vi "Global_Sensors.vi"() -> ()   [LabVIEW 2018]
panel:
  in  "Distance Along Path":dbl
  out "Sensor 1":bool
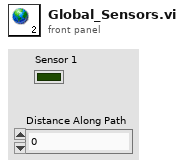
[diagram p1: front panel]
diagram:
